vi "32xx_Décod_Réponse_V_mV_A_mA.vi"(8 "entrée d'erreur":errorcluster caption="entrée d'erreur (pas d'erreur)", 10 "Chaîne\nd'entrée":string="0 OK 12171\r" caption="Chaîne d'entrée", 11 "Visa In":refnum<visa-resource-name>="COM9" caption="Port d'entrée") -> (0 "sortie d'erreur":errorcluster, 1 "Sortie (mV) / (mA)":dbl=12171.0, 2 "Sortie (V) / (A)":dbl=12.171, 3 "Visa Out":refnum<visa-resource-name>="COM9" caption="Port de sortie", 4 "Fin message":bool)   [LabVIEW 2020]
panel:
  # "© 2008 2020 elc  ALL RIGHTS RESERVED."
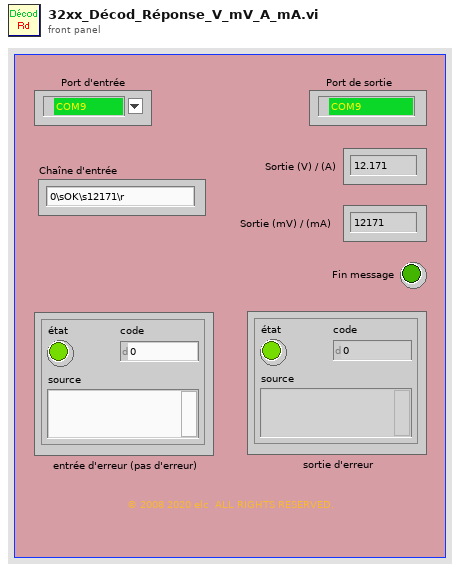
[diagram p1: front panel]
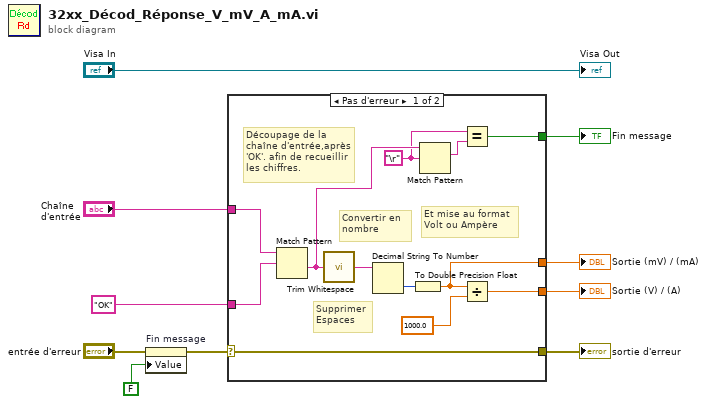
[diagram p0: block diagram]
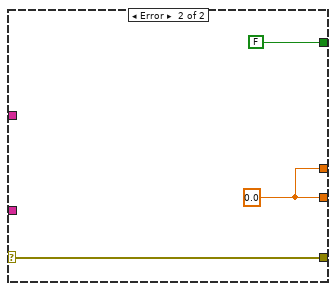
[diagram p2: hidden frame]
diagram:
  n1 = property on="Fin message" class="Bool (strict)"(error in="entrée d'erreur", "Value"=FALSE ("Fin message")) -> (error out=w3:errorcluster)  [unwired: 1 in, 1 out]
  n2 = case shown="Pas d'erreur" w3 {
    selector: w3 -> [w16 w25]
    tunnel: [w17 w23] -> w10
    tunnel: "OK" ("expression régulière") -> [w20 _]
    tunnel: "Chaîne\nd'entrée" -> [w19 _]
    tunnel: [w16 w25] -> w7
    tunnel: [w12 FALSE] -> w6
    tunnel: [w11 w23] -> w5
    frame No Error {
      w13 = "\r" ("expression régulière")
      # "Convertir en \nnombre"
      # "Supprimer\nEspaces"
      # "Et mise au format\nVolt ou Ampère"
      # "Découpage de la chaîne d'entrée,après 'OK'. afin de recueillir les chiffres."
      n3 = Match Pattern(string=w19, regular expression=w20) -> (after substring=w15:string)  [unwired: 1 in, 3 out]
      n4 = call <vilib>:"Trim Whitespace.vi"("string"=w15) -> ("trimmed string"=w21:string)  [unwired: 1 in]
      n5 = Decimal String To Number(string=w21) -> (number=w22:i32)  [unwired: 2 in, 1 out]
      n6 = To Double Precision Float(number=w22) -> (double precision float=w11:dbl)
      n7 = Match Pattern(string=w15, regular expression=w13) -> (match substring=w14:string)  [unwired: 1 in, 3 out]
      n8 = Equal?(x=w13, y=w14) -> (x = y?=w12:bool)
      n9 = Divide(x=w11, y=1000.0) -> (x/y=w17:dbl)
    }
    frame Error {
      w23 = 0.0
    }
  }
  "Sortie (V) / (A)" <- w10
  "sortie d'erreur" <- w7
  "Fin message" <- w6
  "Sortie (mV) / (mA)" <- w5
  "Visa Out" <- "Visa In"
